vi "Write Panes Colors.vi"(8 "error in (no error)":errorcluster, 10 "Colors":T1, 11 "PentaPanesGUI in":refnum<class "PentaPanes.lvclass">) -> (0 "error out":errorcluster, 3 "PentaPanesGUI out":refnum<class "PentaPanes.lvclass">)   [LabVIEW 2022 SP3, in "PentaPanesLibrary.lvlib" / "PentaPanes.lvclass"]
uses:
  PentaPanes.lvclass
  PanesColors.ctl
  PentaPanes.lvclass/PentaPanes.ctl
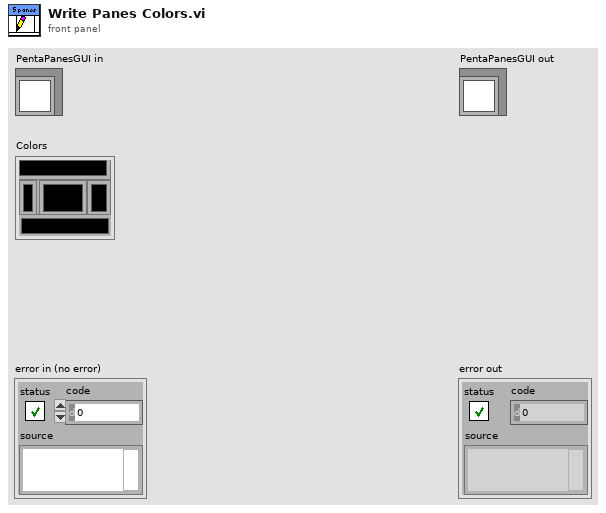
[diagram p1: front panel]
types:
  T1 = typedef "PentaPanesLibrary.lvlib/PentaPanes.lvclass/PanesColors.ctl" = cluster{"Top Color":u32, "Left Color":u32, "Center Color":u32, "Right Color":u32, "Bottom Color":u32}
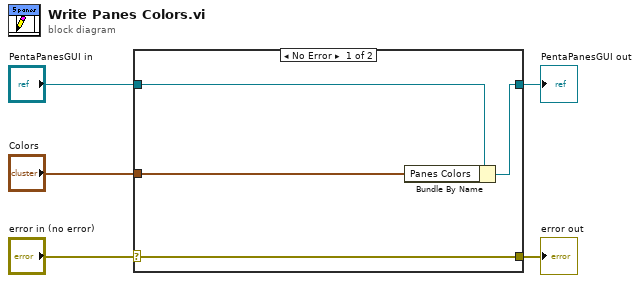
[diagram p0: block diagram]
diagram:
  n1 = case shown="No Error" "error in (no error)" {
    selector: "error in (no error)" -> [w9 w10]
    tunnel: [w9 w10] -> w4
    tunnel: [w7 w11] -> w2
    tunnel: "PentaPanesGUI in" -> [w8 w11]
    tunnel: "Colors" -> [w6 _]
    frame No Error {
      n2 = Bundle By Name(cluster=w8, "Panes Colors"=w6) -> (w7:refnum<class "PentaPanes.lvclass">)
    }
    frame Error {
    }
  }
  "error out" <- w4
  "PentaPanesGUI out" <- w2
